vi "ADC_clean_buffer_batch.vi"(1 "Index":i32, 2 "Readout parameters in":T2(array[cluster]), 3 "Inst_param_in":T1) -> (0 "Readout parameters out":T2(array[cluster]))   [LabVIEW 2013]
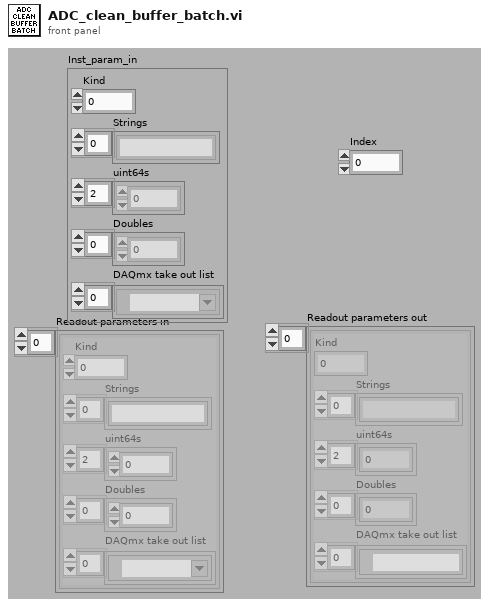
[diagram p1: front panel]
types:
  T1 = cluster{"Kind":u16, "Strings":string[], "uint64s":u64[], "Doubles":dbl[], "DAQmx take out list":refnum<k21>[]}
  T2 = cluster{"Kind":u16, "Strings":string[], "uint64s":u64[], "Doubles":dbl[], "DAQmx take out list":refnum<k21>[]}[]
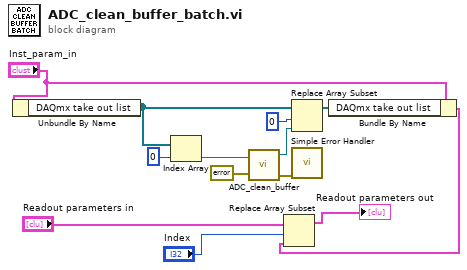
[diagram p0: block diagram]
diagram:
  n1 = Unbundle By Name("Inst_param_in") -> ("DAQmx take out list"=w8:refnum<k21>[])
  n2 = Index Array(array=w8, index=0) -> (element=w10:refnum<k21>)
  n3 = call "ADC_clean_buffer.vi"("error out 2"=errorcluster {"status"=FALSE, "code"=0, "source"=""}, "task out 2"=w10) -> ("error out"=w13:errorcluster, "task out"=w7:refnum<k21>)  [unwired: 1 in]
  n4 = Replace Array Subset(array=w8, new element=w7, index=0) -> (w6:refnum<k21>[])
  n5 = call <vilib>:"Simple Error Handler.vi"("error in (no error)"=w13) -> ()  [unwired: 4 in, 5 out]
  n6 = Bundle By Name(cluster="Inst_param_in", "DAQmx take out list"=w6) -> (w2:T1)
  n7 = Replace Array Subset(array="Readout parameters in", new element=w2, index="Index") -> (→"Readout parameters out":T2)
